vi "Read All Variables.vi"(8 "error in (no error)":errorcluster, 11 "Storage params in":refnum<class "CV-Storage.lvclass">) -> (0 "error out":errorcluster, 2 "Storage vars.":T1, 3 "Storage params out":refnum<class "CV-Storage.lvclass">)   [LabVIEW 2013, in "CameraVision.lvlib" / "CV-Storage.lvclass"]
uses:
  CV-Storage.lvclass
  Storage-variables.ctl
  UI/Module-states.ctl
  CV-Storage.lvclass/CV-Storage.ctl
  UI/CV-UI.lvclass
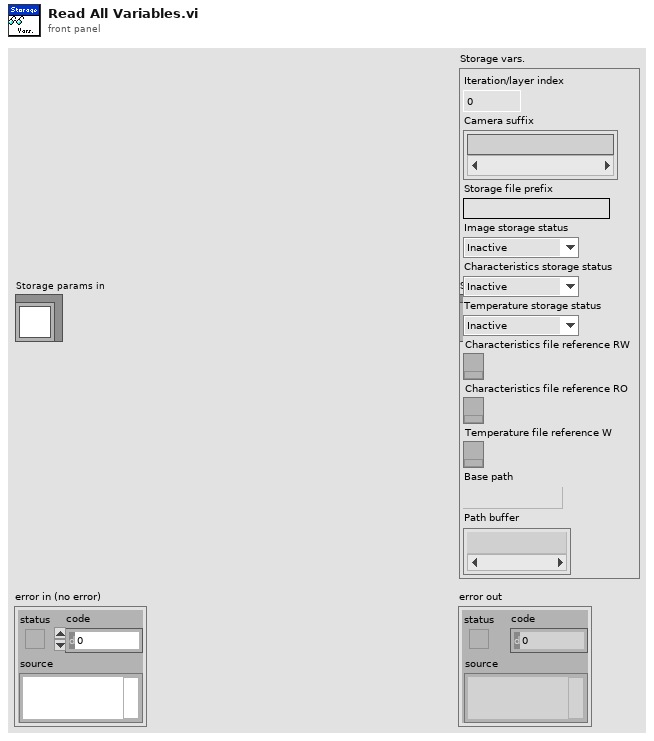
[diagram p1: front panel]
types:
  T1 = typedef "CameraVision.lvlib/CV-Storage.lvclass/Storage-variables.ctl" = cluster{"Iteration/layer index":u16, "Camera suffix":string[], "Storage file prefix":string, "Image storage status":T2, "Characteristics storage status":T2, "Temperature storage status":T2, "Characteristics file reference RW":refnum<k34>, "Characteristics file reference RO":refnum<k34>, "Temperature file reference W":refnum<k34>, "Base path":path, "Path buffer":path[]}
  T2 = typedef "CameraVision.lvlib/CV-UI.lvclass/Module-states.ctl" = enum16{"Inactive", "Active", "Data-loss", "Error", "Simulation", "Synchronizing", "Initialized", "Released"}
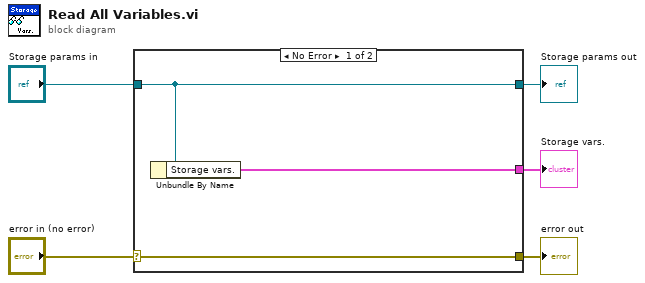
[diagram p0: block diagram]
diagram:
  n1 = case shown="No Error" "error in (no error)" {
    selector: "error in (no error)" -> [w8 w9]
    tunnel: [w8 w9] -> w4
    tunnel: [w7 w10] -> w2
    tunnel: "Storage params in" -> [w7 w10]
    tunnel: [w6 _] -> w1
    frame No Error {
      n2 = Unbundle By Name(w7) -> ("Storage vars."=w6:T1)
    }
    frame Error {
    }
  }
  "error out" <- w4
  "Storage params out" <- w2
  "Storage vars." <- w1
